vi "Stop Control.vi"(11 "Data Cluster":T1) -> ()   [LabVIEW 2020, in "Rotation Stage.lvlib"]
uses:
  Rotation Stage.lvlib
  Module Data--cluster.ctl
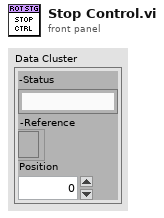
[diagram p1: front panel]
types:
  T1 = typedef "Rotation Stage.lvlib/Module Data--cluster.ctl" = cluster{"-Status":string, "-Reference":refnum<k7>, "Position":sgl}
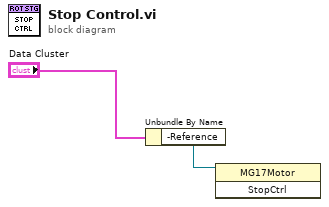
[diagram p0: block diagram]
diagram:
  n1 = Unbundle By Name("Data Cluster") -> ("-Reference"=w2:refnum<k7>)
  n2 = invoke class="MG17Motor" method="StopCtrl"(reference=w2) -> ()  [unwired: 2 in, 3 out]
